vi "Disabled.vi"(7 "Robot Mode":T2, 10 "Match Info":T1={"Autonomous Elapsed Seconds"=0.0, "TeleOp Elapsed Seconds"=0.0, "Disabled Elapsed Seconds"=0.0, "Visited Autonomous"=FALSE, "Visited TeleOp"=FALSE, "Visited Disabled"=FALSE, "Autonomous Settings"={"Autonomous Style"=enum."Independent", "VI Refnum"=refnum}}, 11 "Call Context":T3) -> ()   [LabVIEW 2013]
doc: "This VI is called each time a disabled packet is received from the DS. It is often used to prepare for the next robot mode, to calibrate sensors, etc."
uses:
  <vilib>/Rock Robotics/WPI/DriverStation/WPI_DriverStationDerivedRobotMode.ctl
  <vilib>/Rock Robotics/WPI/DriverStation/WPI_DriverStationRobotMode2.ctl
  <vilib>/Rock Robotics/WPI/DriverStation/WPI_DriverStationMatch Info.ctl
  Robot Global Data.vi
  <vilib>/Rock Robotics/WPI/Joystick/WPI_JoystickGetSetRefNum.vi
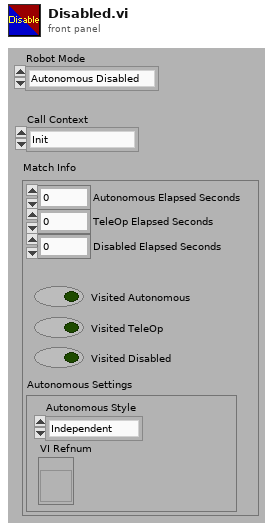
[diagram p1: front panel]
types:
  T1 = typedef "WPI_DriverStationMatch Info.ctl" = cluster{"Autonomous Elapsed Seconds":dbl, "TeleOp Elapsed Seconds":dbl, "Disabled Elapsed Seconds":dbl, "Visited Autonomous":bool, "Visited TeleOp":bool, "Visited Disabled":bool, "Autonomous Settings":cluster{"Autonomous Style":enum16{"Iterative", "Independent"}, "VI Refnum":refnum<vi>}}
  T2 = typedef "WPI_DriverStationRobotMode2.ctl" = enum16{"Autonomous Disabled", "Autonomous Enabled", "Teleop Disabled", "Teleop Enabled", "Timeout", "Finish", "Test Disabled", "Test Enabled"}
  T3 = typedef "WPI_DriverStationDerivedRobotMode.ctl" = enum16{"Init", "Execute", "Stop"}
  T4 = typedef "WPI_JoystickDevRef.ctl" = cluster{"Device":T5}
  T5 = typedef "WPI_JoystickDeviceEnum.ctl" = enum16{"USB 1", "USB 2", "USB 3", "USB 4", "Kinect 1", "Kinect 2"}
  T6 = typedef "WPI_JoystickButtonState.ctl" = cluster{"Button 1":bool, "Button 2":bool, "Button 3":bool, "Button 4":bool, "Button 5":bool, "Button 6":bool, "Button 7":bool, "Button 8":bool, "Button 9":bool, "Button 10":bool, "Button 11":bool, "Button 12":bool}
  T7 = typedef "WPI_MotorControlDeviceRef.ctl" = cluster{"DeviceStatus":errorcluster, "Type":enum16{"PWM", "CAN"}, "PWM":cluster{"Digital Module":T8, "PWM Channel":T9, "DeadBand":T10}, "CAN":cluster{"Device Number":u8, "Control Mode":T11, "Semaphore":T12, "Max Vout":dbl}, "Invert":bool, "TransformRef":T13, "InvTransformRef":T13}
  T8 = typedef "FPGA_TypedefDigitalModule.ctl" = enum16{"Digital Module 1", "Digital Module 2"}
  T9 = typedef "FPGA_DIOPWMChannel.ctl" = enum8{"PWM 1", "PWM 2", "PWM 3", "PWM 4", "PWM 5", "PWM 6", "PWM 7", "PWM 8", "PWM 9", "PWM 10", "Invalid"}
  T10 = typedef "WPI_PWMDeadband.ctl" = cluster{"Name":string, "maxPositivePwm":i32, "minPositivePwm":i32, "centerPwm":i32, "maxNegativePwm":i32, "minNegativePwm":i32, "angularRange":u16}
  T11 = typedef "WPI_CANJaguar_ControlMode.ctl" = enum8{"Percent VBus", "Current", "Speed", "Position", "Voltage"}
  T12 = typedef "Semaphore RefNum" = refnum<k1>
  T13 = typedef "WPI_PWMTransform_ConPane.ctl" = refnum<vi>
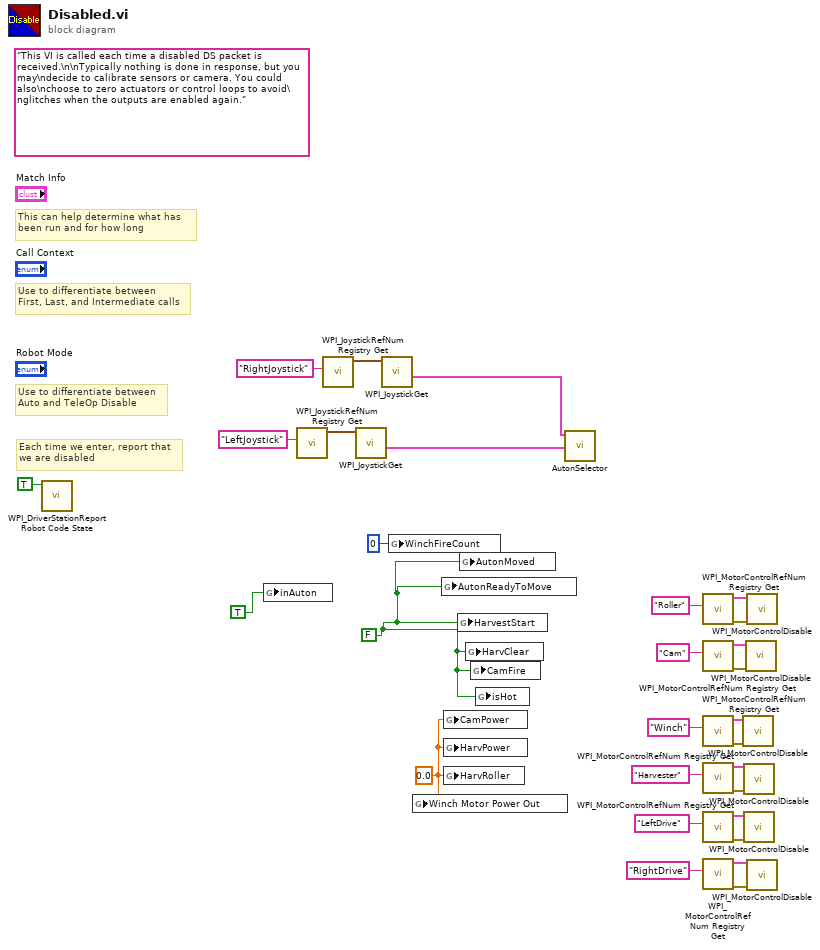
[diagram p0: block diagram]
diagram:
  w4 = 0.0 ("CamPower")
  w1 = FALSE
  (unwired) "This VI is called each time a disabled DS packet is received.\n\nTypically nothing is done in response, but you may\ndecide to calibrate sensors or camera. You could also\nchoose to zero actuators or control loops to avoid\nglitches when the outputs are enabled again."
  # "Each time we enter, report that\nwe are disabled"
  # "Use to differentiate between\nFirst, Last, and Intermediate calls"
  # "This can help determine what has\nbeen run and for how long"
  # "Use to differentiate between\nAuto and TeleOp Disable"
  n1 = call <vilib>:"WPI_DriverStationReport Robot Code State.vi"("Disabled"=TRUE ("Autonomous")) -> ()  [unwired: 10 in, 1 out]
  n2 = global write "Robot Global Data.vi" "inAuton"(TRUE ("inAuton")) -> ()
  n3 = call <vilib>:"WPI_JoystickRefNum Registry Get.vi"("refnum name"="LeftJoystick") -> ("JoystickDevRef"=w24:T4)  [unwired: 9 in, 1 out]
  n4 = call <vilib>:"WPI_JoystickRefNum Registry Get.vi"("refnum name"="RightJoystick") -> ("JoystickDevRef"=w27:T4)  [unwired: 9 in, 1 out]
  n5 = call <vilib>:"WPI_JoystickGet.vi"("JoystickDevRef"=w24) -> ("Buttons"=w23:T6)  [unwired: 4 in, 2 out]
  n6 = call <vilib>:"WPI_JoystickGet.vi"("JoystickDevRef"=w27) -> ("Buttons"=w26:T6)  [unwired: 4 in, 2 out]
  n7 = global write "Robot Global Data.vi" "WinchFireCount"(0 ("WinchFireCount")) -> ()
  n8 = global write "Robot Global Data.vi" "Winch Motor Power Out"(w4) -> ()
  n9 = global write "Robot Global Data.vi" "AutonReadyToMove"(w1) -> ()
  n10 = global write "Robot Global Data.vi" "CamPower"(w4) -> ()
  n11 = global write "Robot Global Data.vi" "HarvPower"(w4) -> ()
  n12 = global write "Robot Global Data.vi" "HarvRoller"(w4) -> ()
  n13 = global write "Robot Global Data.vi" "HarvestStart"(w1) -> ()
  n14 = global write "Robot Global Data.vi" "AutonMoved"(w1) -> ()
  n15 = global write "Robot Global Data.vi" "HarvClear"(w1) -> ()
  n16 = global write "Robot Global Data.vi" "CamFire"(w1) -> ()
  n17 = global write "Robot Global Data.vi" "isHot"(w1) -> ()
  n18 = call "AutonSelector.vi"("Buttons1"=w23, "Buttons in"=w26) -> ()  [unwired: 10 in]
  n19 = call <vilib>:"WPI_MotorControlRefNum Registry Get.vi"("refnum name"="Roller") -> ("error out"=w16:errorcluster, "MotorControlDevRef"=w15:T7)  [unwired: 9 in]
  n20 = call <vilib>:"WPI_MotorControlRefNum Registry Get.vi"("refnum name"="Cam") -> ("error out"=w14:errorcluster, "MotorControlDevRef"=w13:T7)  [unwired: 9 in]
  n21 = call <vilib>:"WPI_MotorControlRefNum Registry Get.vi"("refnum name"="Winch") -> ("error out"=w12:errorcluster, "MotorControlDevRef"=w11:T7)  [unwired: 9 in]
  n22 = call <vilib>:"WPI_MotorControlRefNum Registry Get.vi"("refnum name"="Harvester") -> ("error out"=w10:errorcluster, "MotorControlDevRef"=w9:T7)  [unwired: 9 in]
  n23 = call <vilib>:"WPI_MotorControlRefNum Registry Get.vi"("refnum name"="LeftDrive") -> ("error out"=w8:errorcluster, "MotorControlDevRef"=w7:T7)  [unwired: 9 in]
  n24 = call <vilib>:"WPI_MotorControlRefNum Registry Get.vi"("refnum name"="RightDrive") -> ("error out"=w6:errorcluster, "MotorControlDevRef"=w5:T7)  [unwired: 9 in]
  n25 = call <vilib>:"WPI_MotorControlDisable.vi"("error in (no error)"=w12, "MotorControlDevRef"=w11) -> ()  [unwired: 8 in, 2 out]
  n26 = call <vilib>:"WPI_MotorControlDisable.vi"("error in (no error)"=w10, "MotorControlDevRef"=w9) -> ()  [unwired: 8 in, 2 out]
  n27 = call <vilib>:"WPI_MotorControlDisable.vi"("error in (no error)"=w8, "MotorControlDevRef"=w7) -> ()  [unwired: 8 in, 2 out]
  n28 = call <vilib>:"WPI_MotorControlDisable.vi"("error in (no error)"=w14, "MotorControlDevRef"=w13) -> ()  [unwired: 8 in, 2 out]
  n29 = call <vilib>:"WPI_MotorControlDisable.vi"("error in (no error)"=w16, "MotorControlDevRef"=w15) -> ()  [unwired: 8 in, 2 out]
  n30 = call <vilib>:"WPI_MotorControlDisable.vi"("error in (no error)"=w6, "MotorControlDevRef"=w5) -> ()  [unwired: 8 in, 2 out]
